vi "EEG.vi"() -> ()   [LabVIEW 2019]
uses:
  <vilib>/addons/Biomedical/Controls/Biosignal/Biosignal Spectrum/Biosignal Spectrum.xctl
  <vilib>/addons/Biomedical/Biosignal Measurements/EEG/EEG FFT Spectrum (Waveform).vi
  <vilib>/addons/Biomedical/NI_BMTK_Measurements.lvlib
  <vilib>/addons/Biomedical/NI_BMTK_Controls.lvlib
panel:
  out "EEG Spectrum":cluster{"f0":dbl, "df":dbl, "S(f)":dbl[]}(xcontrol)
  out "beta [%]":dbl
  out "alpha [%]":dbl
  out "theta [%]":dbl
  out "delta [%]":dbl
  out "beta power":dbl
  out "alpha power":dbl
  out "theta power":dbl
  out "delta power":dbl
  in  "stop":bool
  out "Waveform Chart":dynamicdata(graph)
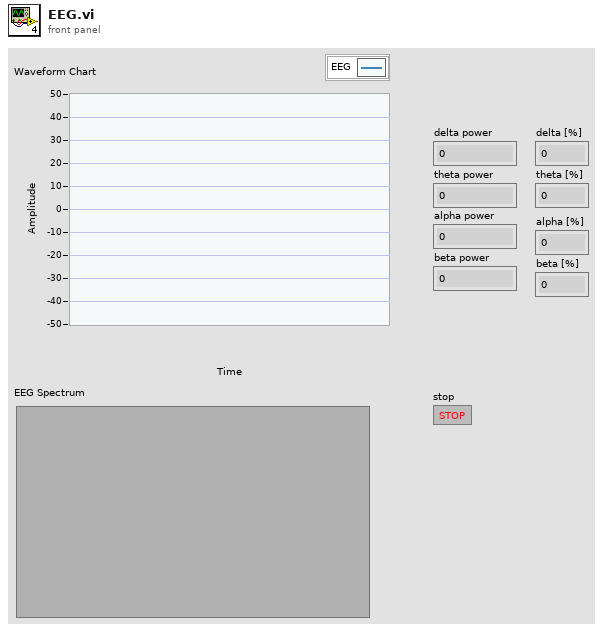
[diagram p1: front panel]
types:
  T1 = typedef "NI_BMTK_Measurements.lvlib/bmt_EEG Frequency-domain Measures.ctl" = cluster{"delta power":dbl, "theta power":dbl, "alpha power":dbl, "beta power":dbl, "delta [%]":dbl, "theta [%]":dbl, "alpha [%]":dbl, "beta [%]":dbl}
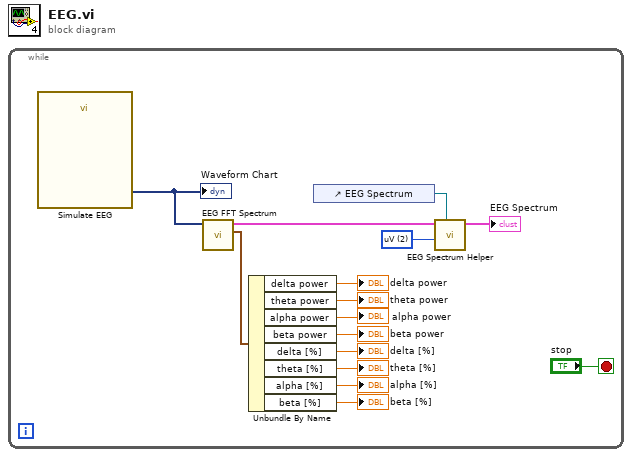
[diagram p0: block diagram]
diagram:
  n1 = while {
    stop <- "stop" stop-if-true
    w2 = u16 2 items=["V", "mV", "uV"] ("RR unit")
    n2 = call "Simulate EEG"() -> ("EEG"=w14:dynamicdata)  [unwired: 10 in, 1 out]
    "Waveform Chart" <- w14
    n3 = call-poly <vilib>:"EEG FFT Spectrum.vi"("EEG"=w14) -> ("frequency measurements"=w13:T1, "FFT spectrum"=w1:cluster{"f0":dbl, "df":dbl, "S(f)":dbl[]})  [unwired: 8 in, 1 out]
    n4 = Unbundle By Name(w13) -> ("delta power"=→"delta power":dbl, "theta power"=→"theta power":dbl, "alpha power"=→"alpha power":dbl, "beta power"=→"beta power":dbl, "delta [%]"=→"delta [%]":dbl, "theta [%]"=→"theta [%]":dbl, "alpha [%]"=→"alpha [%]":dbl, "beta [%]"=→"beta [%]":dbl)
    n5 = control-ref of="EEG Spectrum"() -> (w3:refnum<vi>)
    n6 = call <vilib>:"EEG Spectrum Helper.vi"("EEG spectrum"=w3, "EEG unit"=w2, "spectrum in"=w1) -> ("spectrum out"=→"EEG Spectrum":cluster{"f0":dbl, "df":dbl, "S(f)":dbl[]})  [unwired: 7 in, 1 out]
  }
